vi "Execute Python Optimization (Resync).vi"(8 "error in":errorcluster, 11 "Resynchronization in":refnum<class "Resynchronization.lvclass">) -> (0 "error out":errorcluster, 3 "Resynchronization out":refnum<class "Resynchronization.lvclass">)   [LabVIEW 2018, in "Resynchronization Actor.lvlib" / "Resynchronization.lvclass"]
uses:
  Resynchronization.lvclass
  C:/Users/Administrator/Desktop/LabVIEW EMS/Optimization/Generic Optimization Actor/Generic Optimization/Generic Optimization.lvclass
  Generic Optimization Actor/Generic Optimization/Controls/Grid State for Optimization.ctl
  Global Variables/Global Variables.vi
  Generic Optimization Actor/Generic Optimization/Generic Optimization.lvclass
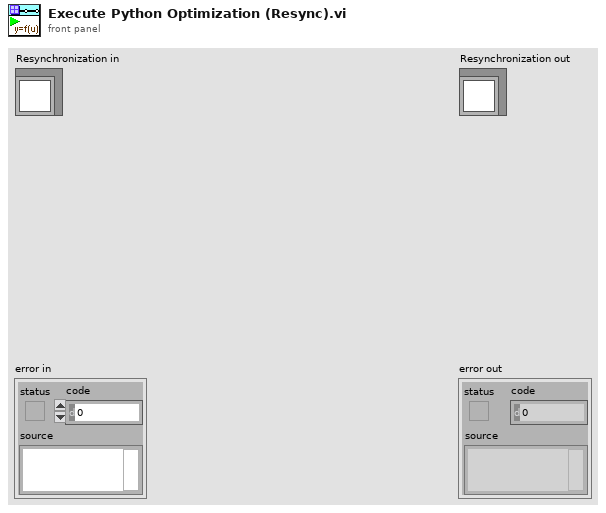
[diagram p1: front panel]
types:
  T1 = typedef "Generic Optimization Actor.lvlib/Generic Optimization.lvclass/Grid State for Optimization.ctl" = enum16{"Invalid", "On-Grid", "Off-Grid", "Island", "Resynch", "Blackstart", "Networked"}
  T2 = typedef "Optimization Type Selector.ctl" = enum16{"Invalid", "Single Phase", "Volttron"}
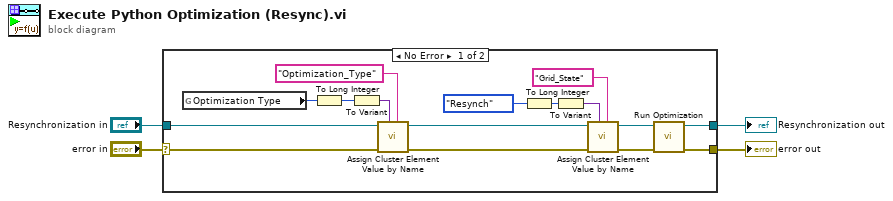
[diagram p0: block diagram]
diagram:
  n1 = case shown="No Error" "error in" {
    selector: "error in" -> [w12 w22]
    tunnel: [w5 w22] -> w1
    tunnel: [w6 w21] -> w3
    tunnel: "Resynchronization in" -> [w9 w21]
    frame No Error {
      n2 = global read "Global Variables.vi" "Optimization Type"() -> (w14:T2)
      n3 = To Long Integer(number=w14) -> (32bit integer=w13:i32)
      n4 = To Variant(anything=w13) -> (Variant=w15:variant)
      n5 = call "Assign Cluster Element Value by Name.vi"("Element Name"="Optimization_Type" ("Keyword Name"), "Value"=w15, "error in"=w12, "Generic Optimization"=w9) -> ("error out"=w11:errorcluster, "Generic Optimization out"=w10:refnum<class "Resynchronization.lvclass">)  [unwired: 6 in]
      n6 = To Long Integer(number=Grid_State_for_Optimization."Resynch") -> (32bit integer=w17:i32)
      n7 = To Variant(anything=w17) -> (Variant=w19:variant)
      n8 = call "Assign Cluster Element Value by Name.vi"("Element Name"="Grid_State" ("Keyword Name"), "Value"=w19, "error in"=w11, "Generic Optimization"=w10) -> ("error out"=w7:errorcluster, "Generic Optimization out"=w8:refnum<class "Resynchronization.lvclass">)  [unwired: 6 in]
      n9 = call "Run Optimization.vi"("error in"=w7, "Generic Optimization"=w8) -> ("error out"=w5:errorcluster, "Generic Optimization out"=w6:refnum<class "Resynchronization.lvclass">)  [unwired: 8 in]
    }
    frame Error {
    }
  }
  "error out" <- w1
  "Resynchronization out" <- w3
